vi "DAQmx_voltage_input_autorange.vi"(8 "error in (no error)":errorcluster, 11 "DAQ task Voltage in":refnum<k21>) -> (0 "error out":errorcluster, 2 "data":dbl, 3 "task out":refnum<k21>, 4 "AI.Max":dbl, 6 "AI.Min":dbl)   [LabVIEW 2017]
uses:
  <vilib>/DAQmx/read.llb/DAQmx Read (Analog DBL 1Chan 1Samp).vi
  <vilib>/DAQmx/miscellaneous.llb/DAQmx Fill In Error Info.vi
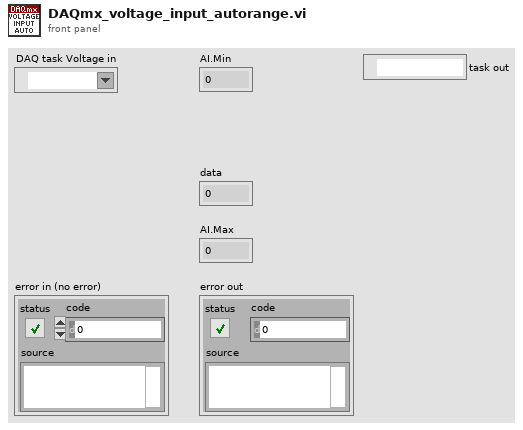
[diagram p1: front panel]
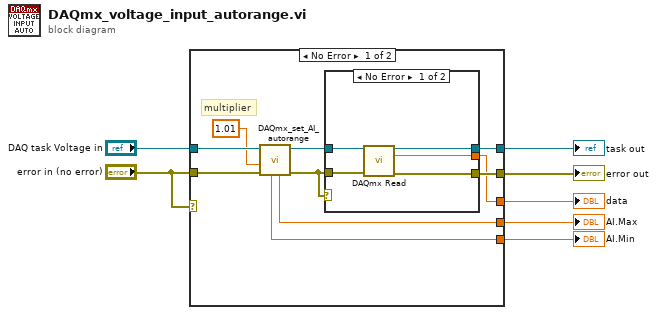
[diagram p0: block diagram]
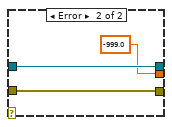
[diagram p2: hidden frame]
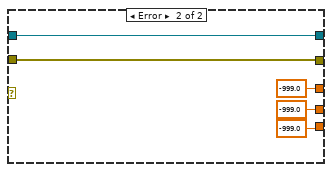
[diagram p3: hidden frame]
diagram:
  n1 = case shown="No Error" "error in (no error)" {
    tunnel: "DAQ task Voltage in" -> [w17 w30]
    tunnel: [w9 -999.0 ("AI.Min")] -> w6
    tunnel: [w8 -999.0 ("AI.Max")] -> w5
    tunnel: [w16 w29] -> w4
    tunnel: "error in (no error)" -> [w13 w29]
    tunnel: [w12 -999.0 ("data")] -> w3
    tunnel: [w11 w30] -> w2
    frame No Error {
      # "multiplier"
      n2 = call "DAQmx_set_AI_autorange.vi"("error in (no error)"=w13, "multiplier"=1.01, "task/channels in"=w17) -> ("error out"=w10:errorcluster, "task out"=w14:refnum<k21>, "AI.Max"=w8:dbl, "AI.Min"=w9:dbl)  [unwired: 5 in]
      n3 = case shown="No Error" w10 {
        tunnel: [w22 w24] -> w16
        tunnel: w10 -> [w21 w24]
        tunnel: w14 -> [w20 w25]
        tunnel: [w19 -999.0 ("data")] -> w12
        tunnel: [w18 w25] -> w11
        frame No Error {
          n4 = call-poly <vilib>:"DAQmx Read.vi"("task/channels in"=w20, "error in"=w21) -> ("task out"=w18:refnum<k21>, "data"=w19:dbl, "error out"=w22:errorcluster)  [unwired: 11 in]
        }
        frame Error {
        }
      }
    }
    frame Error {
    }
  }
  "AI.Min" <- w6
  "AI.Max" <- w5
  "error out" <- w4
  "data" <- w3
  "task out" <- w2
